vi "Convert VeriStand Variant.vi"(8 "error in (no error)":errorcluster, 10 "Data":u8[](array[numeric]), 11 "Type array":u8[](array[numeric])) -> (0 "error out":errorcluster, 3 "Variant":variant)   [LabVIEW 2015, in "J1939 Workspace Object.lvlib"]
uses:
  J1939 Workspace Object.lvlib
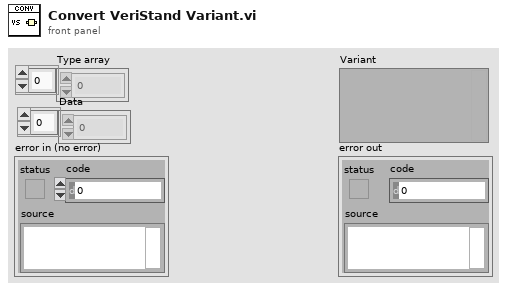
[diagram p1: front panel]
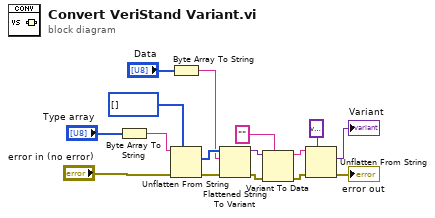
[diagram p0: block diagram]
diagram:
  n1 = Byte Array To String(unsigned byte array="Type array") -> (string=w13:string)
  n2 = Byte Array To String(unsigned byte array="Data") -> (string=w12:string)
  n3 = Unflatten From String(type=i16[] [] ("type string"), binary string=w13, error in (no error)="error in (no error)") -> (value=w15:i16[], error out=w14:errorcluster)  [unwired: 2 in, 1 out]
  n4 = Flattened String To Variant(4:w14, 6:w12, 7:w15) -> (0:w8:errorcluster, 3:w11:variant)
  n5 = Variant To Data(error in=w8, type="", Variant=w11) -> (data=w9:string, error out=w7:errorcluster)
  n6 = Unflatten From String(type=variant ("variant"), binary string=w9, error in (no error)=w7) -> (value=→"Variant":variant, error out=→"error out":errorcluster)  [unwired: 2 in, 1 out]
